vi "GetScriptName.vi"(8 "error in":errorcluster, 11 "ConfigINIFiles":path[](array[path])) -> (0 "error out":errorcluster, 3 "Script Names":string[](array[string]))   [LabVIEW 2018, in "Test.lvclass"]
doc: "This VI retrieves all the section names in the INI file(s)."
uses:
  Test.lvclass
  <vilib>/Utility/config.llb/NI_LVConfig.lvlib
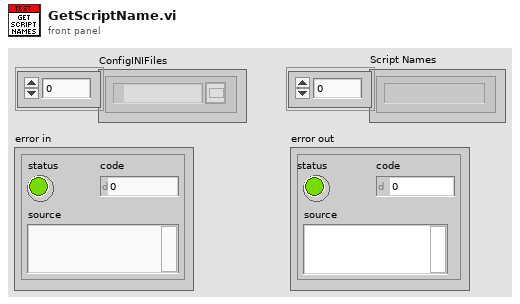
[diagram p1: front panel]
types:
  T1 = typedef "NI_LVConfig.lvlib/Config Data RefNum.ctl" = refnum<k1>
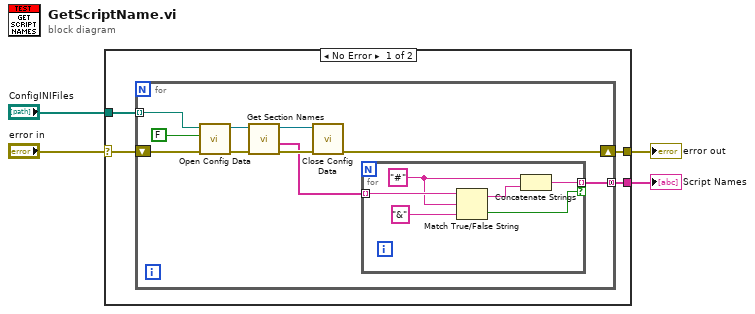
[diagram p0: block diagram]
diagram:
  n1 = case shown="No Error" "error in" {
    selector: "error in" -> [w8 w25]
    tunnel: [w7 w25] -> w1
    tunnel: "ConfigINIFiles" -> [w6 _]
    tunnel: [w5 _] -> w3
    frame No Error {
      n2 = for {
        shift-right: [w17] -> w7
        shift-left: w8 -> [w18]
        tunnel: w6 -> [w15] mode=indexing
        tunnel: [w9] -> w5 mode=concatenating
        n3 = call <vilib>:"Open Config Data.vi"("error in (no error)"=w18, "create file if necessary (T)"=FALSE, "configuration file path"=w15) -> ("error out"=w13:errorcluster, "refnum"=w14:T1)  [unwired: 6 in, 1 out]
        n4 = call <vilib>:"Get Section Names.vi"("error in (no error)"=w13, "refnum"=w14) -> ("error out"=w12:errorcluster, "section names"=w10:string[], "refnum out"=w11:T1)  [unwired: 7 in]
        n5 = call <vilib>:"Close Config Data.vi"("error in (no error)"=w12, "refnum"=w11) -> ("error out"=w17:errorcluster)  [unwired: 8 in, 1 out]
        n6 = for {
          tunnel: w10 -> [w24] mode=indexing
          tunnel: [w19] -> w9 mode=indexing if=w23
          w20 = "#" ("true string")
          n7 = Match True/False String(2:"&" ("false string"), 3:w20, 4:w24) -> (0:w23:bool, 1:w21:string)
          n8 = Concatenate Strings(w20, w21) -> (w19:string)
        }
      }
    }
    frame Error {
    }
  }
  "error out" <- w1
  "Script Names" <- w3
